vi "Write High Alarm Limit.vi"(8 "error in (no error)":errorcluster, 10 "High Alarm Limit":variant, 11 "NT Scalar (Numeric) in":refnum<class "NT Scalar (Numeric).lvclass">) -> (0 "error out":errorcluster, 3 "NT Scalar (Numeric) out":refnum<class "NT Scalar (Numeric).lvclass">)   [LabVIEW 2020, in "PV Access.lvlib" / "PV Data.lvlib" / "NT Scalar (Numeric).lvclass"]
uses:
  NT Scalar (Numeric).lvclass
  NT Scalar (Numeric).lvclass/NT Scalar (Numeric).ctl
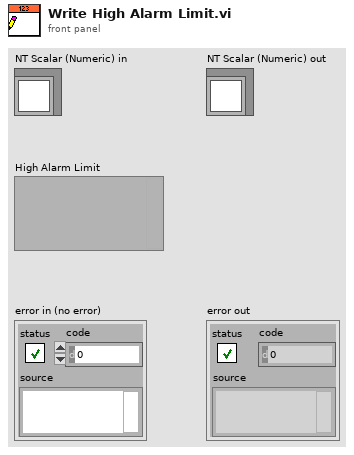
[diagram p1: front panel]
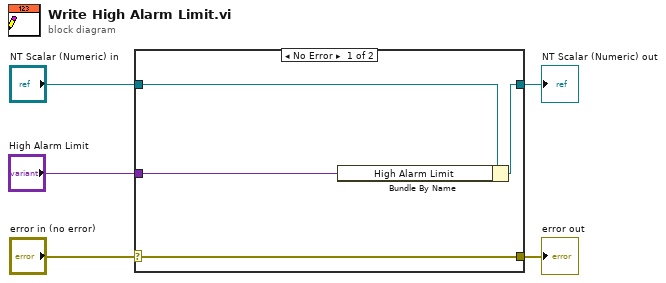
[diagram p0: block diagram]
diagram:
  n1 = case shown="No Error" "error in (no error)" {
    selector: "error in (no error)" -> [w9 w10]
    tunnel: [w9 w10] -> w4
    tunnel: [w7 w11] -> w2
    tunnel: "NT Scalar (Numeric) in" -> [w8 w11]
    tunnel: "High Alarm Limit" -> [w6 _]
    frame No Error {
      n2 = Bundle By Name(cluster=w8, "High Alarm Limit"=w6) -> (w7:refnum<class "NT Scalar (Numeric).lvclass">)
    }
    frame Error {
    }
  }
  "error out" <- w4
  "NT Scalar (Numeric) out" <- w2
